vi "JC_IG4500_run.vi"(0 "VISA IN":refnum<visa-resource-name>, 5 "Fil on":bool, 7 "Fil off":bool, 9 "Degas on":bool, 11 "Degas off":bool) -> (4 "Readback array":string[](array[string]), 15 "Error Message":string=" INSTRUCTIONS:\r\rNormal Use:  When using subVIs that incorporate the error in/error out (or error I/O) structure, place this handler where you want to inform the user of an error, typically at the end of the I/O data path, as the last action of the program.  If the error in error? is ERROR, the handler creates a message describing the error and its source.  If the type of dialog = 1 (default), the message is displayed to the user, who can only acknowedge it.  If the type = 2, the user can acknowledge the message or abort execution; aborting a program with active I/O is not recommended.  If the type = 0, no message is displayed; this is used to process the error programmatically, and the error out cluster elements are wired to individual terminals for that reason.  \r\rOther Use:\n\r\nlocal testing.  To test the error code of a subVI or function that does not have the error I/O structure, you can wire its error code and a source string to the local error code and error source inputs.  If error in error? indicates no error and error code is not equal to 0, the local code and source are substituted for the error in values, and error? is set TRUE (ERROR).")   [LabVIEW 2013]
panel:
  out "Commands being sent":string[](array[string])
  in  "SD0":string="=SD0"
  in  "SD1":string="=SD1"
  in  "SF0":string="=SF0"
  in  "SF1":string="=SF1"
  out "read buffer":string
  out "Ascii Vacuum Reading":string
  # "Additional Commands"
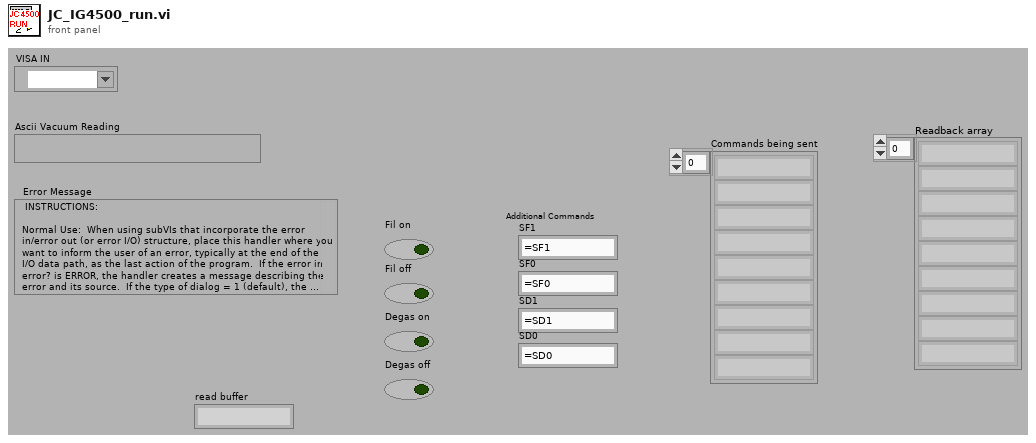
[diagram p1: front panel]
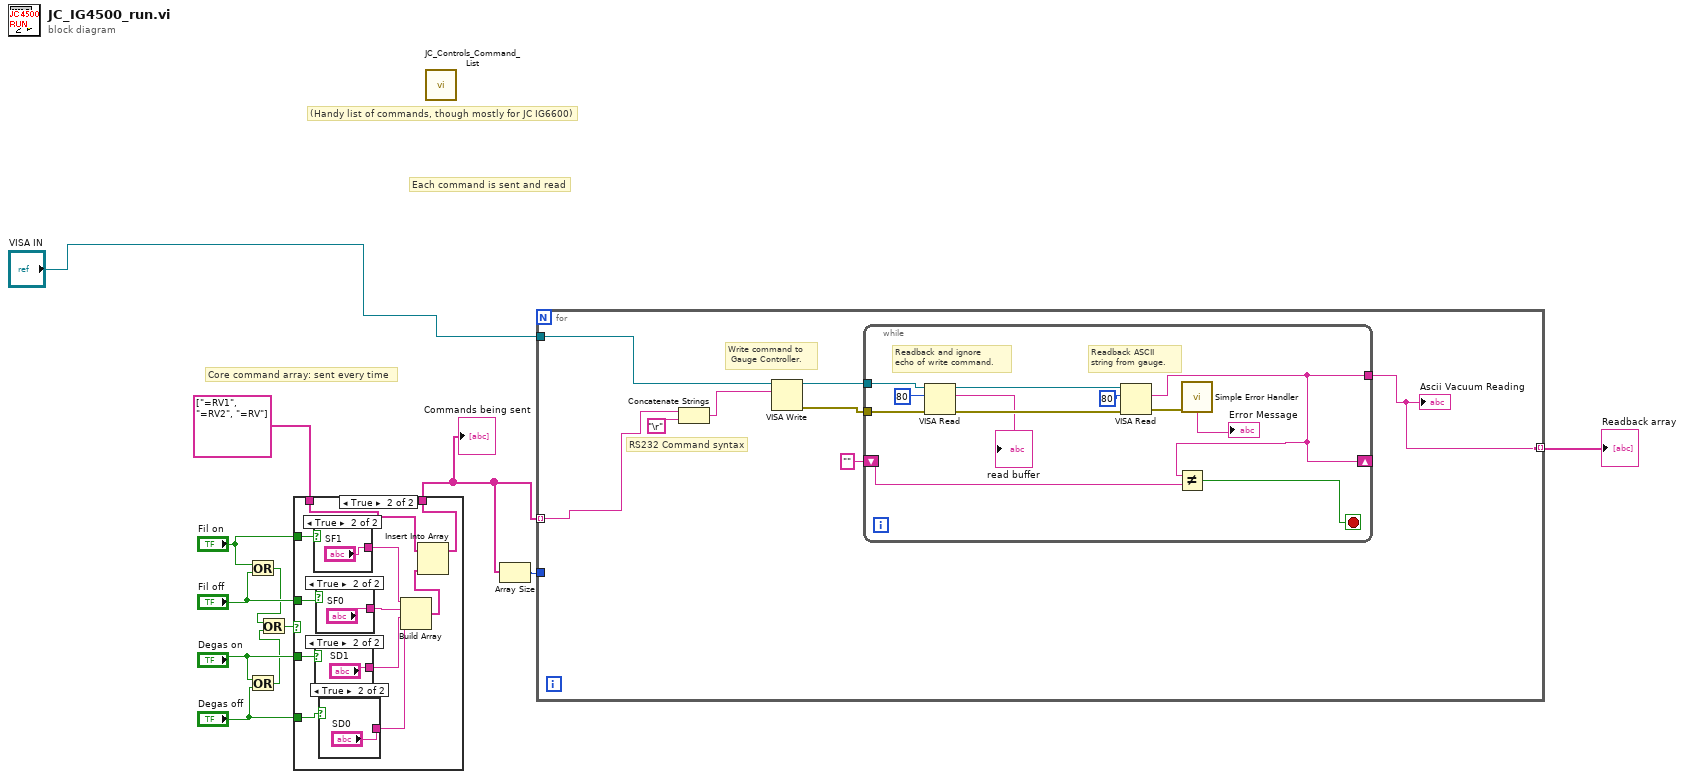
[diagram p0: block diagram]
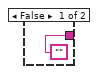
[diagram p3: hidden frame]
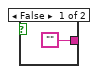
[diagram p4: hidden frame]
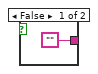
[diagram p5: hidden frame]
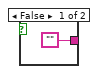
[diagram p6: hidden frame]
diagram:
  # "Core command array: sent every time"
  # "Each command is sent and read"
  # "(Handy list of commands, though mostly for JC IG6600)"
  n1 = Or(x="Fil on", y="Fil off") -> (x .or. y?=w6:bool)
  n2 = Or(x="Degas on", y="Degas off") -> (x .or. y?=w5:bool)
  n3 = Or(x=w6, y=w5) -> (x .or. y?=w4:bool)
  n4 = case shown="True" w4 {
    tunnel: "Fil on" -> [_ w24]
    tunnel: "Fil off" -> [_ w22]
    tunnel: "Degas on" -> [_ w21]
    tunnel: "Degas off" -> [_ w20]
    tunnel: string[] ["=RV1", "=RV2", "=RV"] ("Commands being sent 2") -> [w13 w15]
    tunnel: [w13 w14] -> w3
    frame False {
    }
    frame True {
      n5 = case shown="True" w24 {
        tunnel: ["" "SF1"] -> w23
        frame False {
        }
        frame True {
        }
      }
      n6 = case shown="True" w21 {
        tunnel: ["" "SD1"] -> w18
        frame False {
        }
        frame True {
        }
      }
      n7 = case shown="True" w22 {
        tunnel: ["" "SF0"] -> w19
        frame False {
        }
        frame True {
        }
      }
      n8 = case shown="True" w20 {
        tunnel: ["" "SD0"] -> w17
        frame False {
        }
        frame True {
        }
      }
      n9 = Build Array(w23, w19, w18, w17) -> (w16:string[])
      n10 = Insert Into Array(array=w15, new element=w16) -> (w14:string[])  [unwired: 1 in]
    }
  }
  "Commands being sent" <- w3
  n11 = call "JC_Controls_Command_List.vi"() -> ()  [unwired: 1 in]
  n12 = Array Size(array=w3) -> (size(s)=w12:i32)
  n13 = for {
    tunnel: "VISA IN" -> [w38]
    tunnel: w3 -> [w34] mode=indexing
    tunnel: w12 -> [_]
    tunnel: [w33] -> w11 mode=indexing
    # "Write command to\n Gauge Controller."
    # "RS232 Command syntax"
    n14 = Concatenate Strings(w34, "\r") -> (w39:string)
    n15 = VISA Write(VISA resource name=w38, write buffer=w39) -> (VISA resource name out=w36:refnum<visa-resource-name>, error out=w37:errorcluster)  [unwired: 1 in, 1 out]
    n16 = while {
      tunnel: w37 -> [w46]
      tunnel: w36 -> [w45]
      shift-right: [w42] -> _
      shift-left: "" ("read buffer") -> [w44]
      tunnel: [w42] -> w33
      stop <- w43 stop-if-true
      # "Readback ASCII\nstring from gauge."
      # "Readback and ignore\necho of write command."
      n17 = VISA Read(VISA resource name=w45, byte count=u32 80 ("Bytes to Read"), error in (no error)=w46) -> (VISA resource name out=w51:refnum<visa-resource-name>, read buffer=→"read buffer":string, error out=w52:errorcluster)  [unwired: 1 out]
      n18 = VISA Read(VISA resource name=w51, byte count=u32 80 ("Bytes to Read"), error in (no error)=w52) -> (read buffer=w42:string, error out=w49:errorcluster)  [unwired: 2 out]
      n19 = Not Equal?(x=w42, y=w44) -> (x != y?=w43:bool)
      n20 = call <vilib>:"Simple Error Handler.vi"("error in (no error)"=w49) -> ("message"=→"Error Message":string)  [unwired: 4 in, 4 out]
    }
    "Ascii Vacuum Reading" <- w33
  }
  "Readback array" <- w11
